vi "Get-values-from-reference.vi"(8 "error in (no error)":errorcluster, 11 "Controls to save in":refnum<vi>[](array[refnum])) -> (0 "error out":errorcluster, 2 "Values":T1(array[cluster]), 3 "Controls to save out":refnum<vi>[](array[refnum]))   [LabVIEW 2013, in "SettingsFile.lvlib" / "SettingsFile.lvclass"]
uses:
  SettingsFile.lvclass
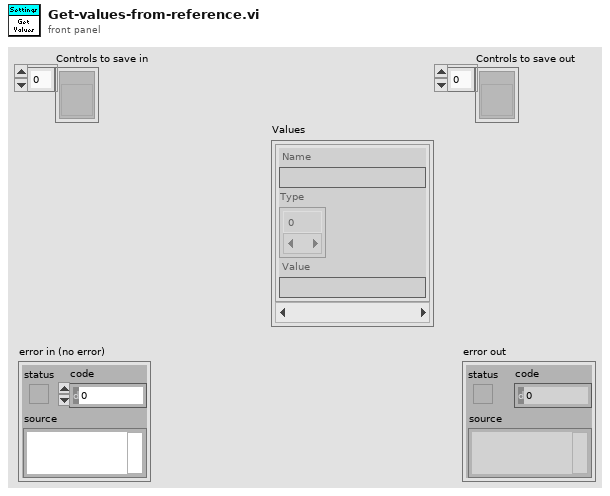
[diagram p1: front panel]
types:
  T1 = cluster{"Name":string, "Type":i16[], "Value":string}[]
  T2 = cluster{"Name":string, "Type":i16[], "Value":string}
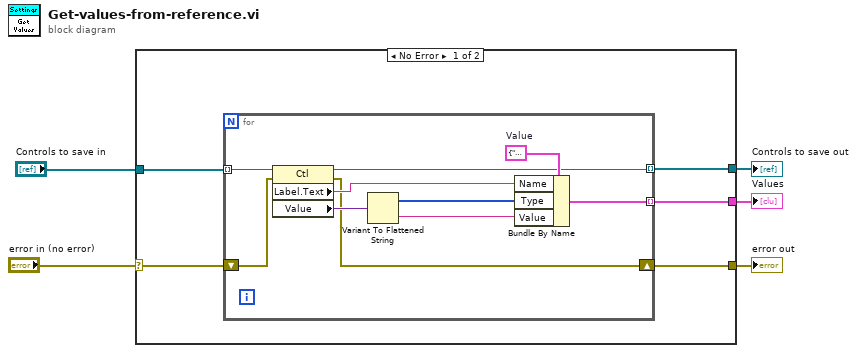
[diagram p0: block diagram]
diagram:
  n1 = case shown="No Error" "error in (no error)" {
    selector: "error in (no error)" -> [w9 w22]
    tunnel: [w7 w22] -> w4
    tunnel: "Controls to save in" -> [w10 w21]
    tunnel: [w8 _] -> w2
    tunnel: [w6 w21] -> w1
    frame No Error {
      n2 = for {
        tunnel: w10 -> [w20] mode=indexing
        shift-right: [w13] -> w7
        shift-left: w9 -> [w12]
        tunnel: [w14] -> w8 mode=indexing
        tunnel: [w11] -> w6 mode=indexing
        w18 = T2 {"Name"="", "Type"=[], "Value"=""}  # Value
        n3 = property class="Ctl"(reference=w20, error in=w12) -> (reference out=w11:refnum<vi>, error out=w13:errorcluster, "Label.Text"=w17:string, "Value"=w19:variant)
        n4 = Variant To Flattened String(Variant=w19) -> (data string=w15:string, 1:w16:i16[])
        n5 = Bundle By Name(cluster=w18, "Name"=w17, "Type"=w16, "Value"=w15) -> (w14:T2)
      }
    }
    frame Error {
    }
  }
  "error out" <- w4
  "Values" <- w2
  "Controls to save out" <- w1
